vi "rad2deg.vi"(1 "rad":dbl) -> (0 "deg":dbl)   [LabVIEW 2011]
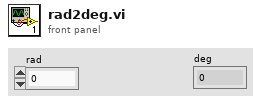
[diagram p1: front panel]
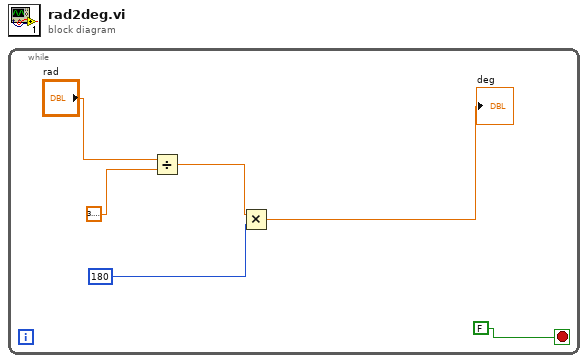
[diagram p0: block diagram]
diagram:
  n1 = while {
    stop <- FALSE stop-if-true
    n2 = Divide(x="rad", y=3.141592653589793) -> (x/y=w4:dbl)
    n3 = Multiply(x=w4, y=180) -> (x*y=→"deg":dbl)
  }
